vi "2 RIO.vi"   [LabVIEW 2011]
uses:
  2 Globals/2 Global.vi
types:
  T1 = typedef "UTM Location.ctl" = cluster{"UTM Zone":dbl, "Hemisphere":enum16{"North", "South"}, "East":dbl, "North":dbl}
  T2 = typedef "Velocity.ctl" = cluster{"East":dbl, "North":dbl}
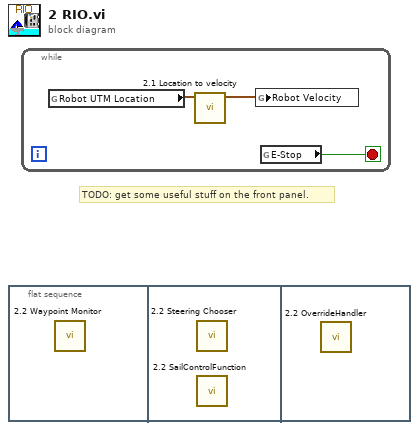
[diagram p0: block diagram]
diagram:
  # "TODO: get some useful stuff on the front panel."
  n1 = flat-sequence {
    frame #0 {
      n2 = call "2.2 Waypoint Monitor.vi"() -> ()  [unwired: 12 in]
    }
    frame #1 {
      n3 = call "2.2 Steering Chooser.vi"() -> ()  [unwired: 12 in]
      n4 = call "2.2 SailControlFunction.vi"() -> ()  [unwired: 12 in]
    }
    frame #2 {
      n5 = call "2.2 OverrideHandler.vi"() -> ()  [unwired: 12 in]
    }
  }
  n6 = while {
    stop <- w1 stop-if-true
    n7 = global read "2 Global.vi" "Robot UTM Location"() -> (w2:T1)
    n8 = call "2.1 Location to velocity.vi"("Robot UTM Location"=w2) -> ("Velocity"=w3:T2)  [unwired: 10 in]
    n9 = global write "2 Global.vi" "Robot Velocity"(w3) -> ()
    n10 = global read "2 Global.vi" "E-Stop"() -> (w1:bool)
  }
